vi "Get Category.vi"(8 "error in (no error)":errorcluster, 11 "GPIC Core editor node in":refnum<class "GPIC Core editor node.lvclass">) -> (0 "error out":errorcluster, 2 "Category":string, 3 "GPIC Core editor node out":refnum<class "GPIC Core editor node.lvclass">)   [LabVIEW 2017, in "GPIC Core editor node.lvclass"]
uses:
  GPIC Core editor node.lvclass
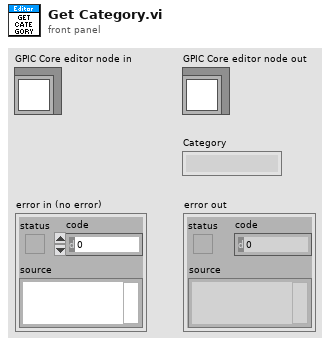
[diagram p1: front panel]
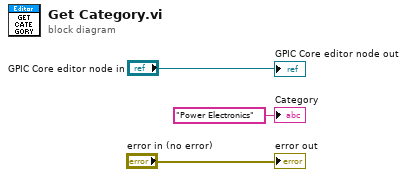
[diagram p0: block diagram]
diagram:
  "error out" <- "error in (no error)"
  "GPIC Core editor node out" <- "GPIC Core editor node in"
  "Category" <- "Power Electronics" ("Category")
